vi "Stop.vi"(8 "error in (no error)":errorcluster, 10 "Message in":refnum<class "StopMessage.lvclass">=refnum, 11 "Cobolt in":refnum<class "Cobolt.lvclass">) -> (0 "error out":errorcluster, 3 "Cobolt out":refnum<class "Cobolt.lvclass">)   [LabVIEW 2012, in "Cobolt.lvclass"]
doc: "This member function is called when the statemachine in the run.vi receives an 'stop' command. It relays the message to all observers of the component.\n\nOverride this member function in your derived class if you need additional stop functionality (but don't forget to call the parent method)."
uses:
  Cobolt.lvclass
  <vilib>/Distrio/Murmex/Murmex/Murmex.lvclass
  Murmex/LabVIEW/Murmex/StopMessage/StopMessage.lvclass
panel:
  # "This method is called when the STOP\ntrigger is sent. \n\nOverride this method when your component needs to\nrespond to this trigger. \n\nCall parent for proper implementation"
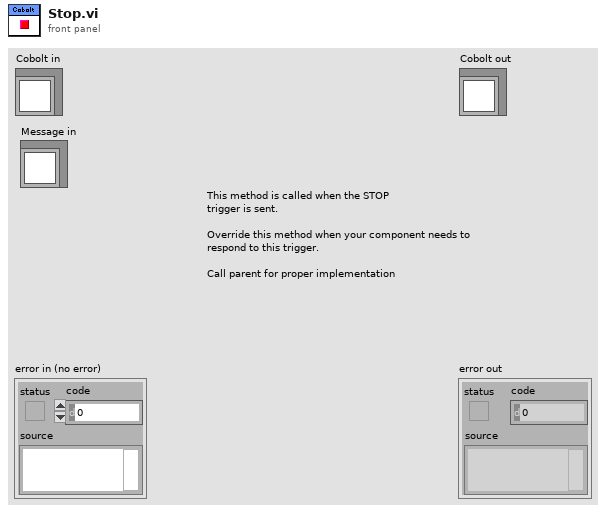
[diagram p1: front panel]
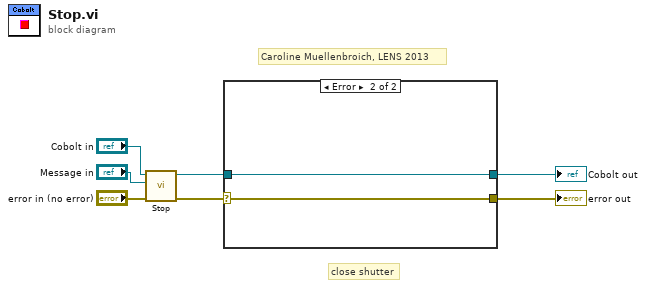
[diagram p0: block diagram]
diagram:
  # "Caroline Muellenbroich, LENS 2013"
  # "close shutter"
  n1 = call-parent "Stop.vi"("error in (no error)"="error in (no error)", "Message in"="Message in", "Murmex in"="Cobolt in") -> ("error out"=w4:errorcluster, "Murmex out"=w2:refnum<class "Cobolt.lvclass">)  [unwired: 7 in]
  n2 = case shown="Error" w4 {
    selector: w4 -> [w9 w11]
    tunnel: [w9 w11] -> w3
    tunnel: w2 -> [w8 w10]
    tunnel: [w8 w10] -> w1
    frame No Error {
    }
    frame Error {
    }
  }
  "error out" <- w3
  "Cobolt out" <- w1
